vi "Cost.vi"(8 "error in (no error)":errorcluster caption="错误输入（无错误）", 11 "Espresso 输入":refnum<class "Espresso.lvclass">) -> (0 "error out":errorcluster caption="错误输出", 2 "cost":dbl, 3 "Espresso 输出":refnum<class "Espresso.lvclass">)   [LabVIEW 2016, in "Espresso.lvclass"]
uses:
  Espresso.lvclass
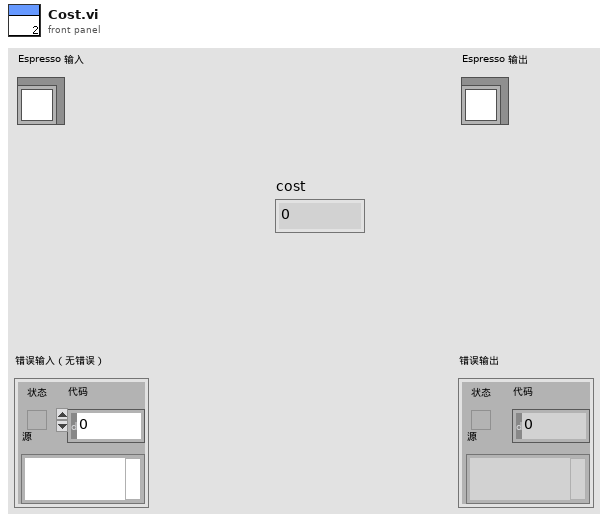
[diagram p1: front panel]
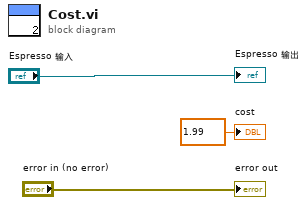
[diagram p0: block diagram]
diagram:
  "error out" <- "error in (no error)"
  "Espresso 输出" <- "Espresso 输入"
  "cost" <- 1.99 ("cost")
